vi "getOrientationOffset.vi"(8 "error in (no error)":errorcluster, 10 "pOffsetTypeStr":string, 11 "pHandle":u32) -> (0 "error out":errorcluster, 2 "return type":i32, 3 "rotationMatrix":sgl[](array[numeric]))   [LabVIEW 2011, in "sbgLabView.lvlib"]
uses:
  sbgLabView.lvlib
  sbgMatLab.dll
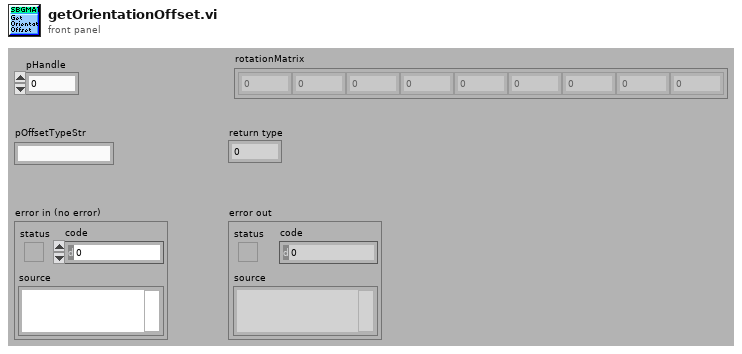
[diagram p1: front panel]
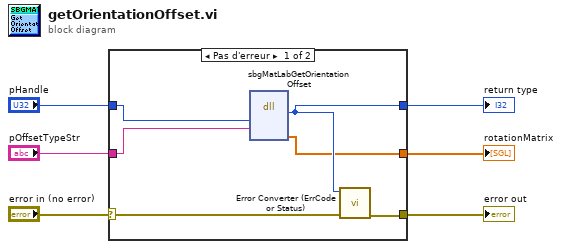
[diagram p0: block diagram]
diagram:
  n1 = case shown="Pas d'erreur" "error in (no error)" {
    selector: "error in (no error)" -> [w8 w13]
    tunnel: [w7 w13] -> w5
    tunnel: [w12 _] -> w4
    tunnel: "pHandle" -> [w11 _]
    tunnel: "pOffsetTypeStr" -> [w10 _]
    tunnel: [w9 _] -> w1
    frame No Error {
      n2 = dll-call lib="C:/SBG-Systems/remote/projects/software/projects/labviewExample/sbgLabView/sbgMatLab.*" fn="sbgMatLabGetOrientationOffset"("pHandle"=w11, "offsetTypeStr"=w10) -> ("return type"=w12:i32, "rotationMatrix"=w9:sgl[])  [unwired: 6 in, 2 out]
      n3 = call "Error Converter (ErrCode or Status).vi"("error in (no error)"=w8, "error code"=w12) -> ("error out"=w7:errorcluster)  [unwired: 9 in]
    }
    frame Error {
    }
  }
  "return type" <- w4
  "rotationMatrix" <- w1
  "error out" <- w5
